vi "Configure Baud Rate.vi"(8 "error in (no error)":errorcluster, 10 "baud rate":u32(ring)=19200 items=["300"=300, "600"=600, "1200"=1200, "2400"=2400, "4800"=4800, "9600"=9600, "19200"=19200, "38400"=38400, "76800"=76800, "115200"=115200], 11 "VI Probe in":refnum<class "PL MKS VI Probe.lvclass">) -> (0 "error out":errorcluster, 3 "VI Probe out":refnum<class "PL MKS VI Probe.lvclass">)   [LabVIEW 2015, in "PL MKS VI Probe.lvclass"]
doc: "Configures baud rate."
uses:
  PL MKS VI Probe.lvclass
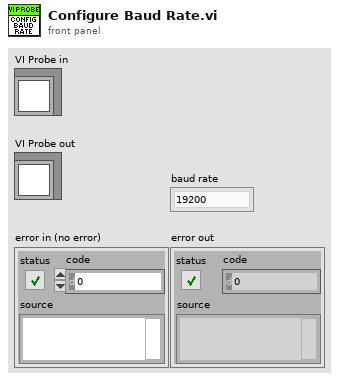
[diagram p1: front panel]
types:
  T1 = typedef "LVStringsAndValuesArrayTypeDef_U32.ctl" = cluster{"String":string, "Value":u32}[]
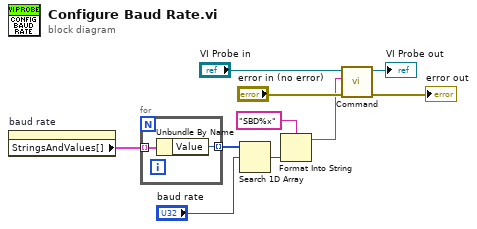
[diagram p0: block diagram]
diagram:
  n1 = property on="baud rate" class="Ring (strict)"() -> ("StringsAndValues[]"=w10:T1)  [unwired: 2 in, 2 out]
  n2 = for {
    tunnel: w10 -> [w12] mode=indexing
    tunnel: [w11] -> w9 mode=indexing
    n3 = Unbundle By Name(w12) -> ("Value"=w11:u32)
  }
  n4 = Search 1D Array(1D array=w9, element="baud rate") -> (index of element=w6:i32)  [unwired: 1 in]
  n5 = Format Into String(format string="SBD%x", w6) -> (resulting string=w1:string)  [unwired: 2 in, 1 out]
  n6 = call "Command.vi"("error in (no error)"="error in (no error)", "command"=w1, "VI Probe in"="VI Probe in") -> ("error out"=→"error out":errorcluster, "VI Probe out"=→"VI Probe out":refnum<class "PL MKS VI Probe.lvclass">)  [unwired: 6 in, 1 out]
